vi "write_erg.vi"(8 "error in (no error)":errorcluster, 9 "byte count":u32, 10 "unsigned byte array":u8[](array[numeric]), 11 "VISA resource name":refnum<visa-resource-name>) -> (0 "error out":errorcluster, 1 "Errors":bool, 2 "unsigned byte array 2":u8[](array[numeric]), 3 "VISA resource name out":refnum<visa-resource-name>)   [LabVIEW 2018]
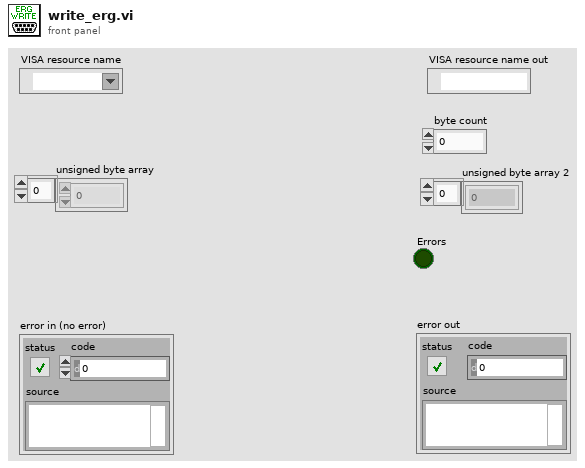
[diagram p1: front panel]
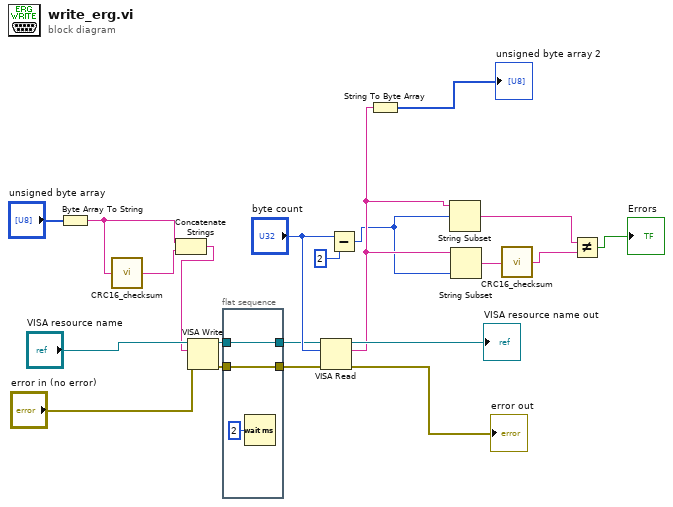
[diagram p0: block diagram]
diagram:
  n1 = Byte Array To String(unsigned byte array="unsigned byte array") -> (string=w17:string)
  n2 = call "CRC16_checksum.vi"("message"=w17) -> ("CRC16"=w16:string)
  n3 = Concatenate Strings(w17, w16) -> (w15:string)
  n4 = VISA Write(VISA resource name="VISA resource name", write buffer=w15, error in (no error)="error in (no error)") -> (VISA resource name out=w4:refnum<visa-resource-name>, error out=w1:errorcluster)  [unwired: 1 out]
  n5 = flat-sequence {
    tunnel: w4 -> [w24]
    tunnel: [w24] -> w3
    tunnel: [w23] -> w2
    tunnel: w1 -> [w23]
    frame #0 {
      n6 = Wait (ms)(milliseconds to wait=u32 2) -> ()  [unwired: 1 out]
    }
  }
  n7 = VISA Read(VISA resource name=w3, byte count="byte count", error in (no error)=w2) -> (VISA resource name out=→"VISA resource name out":refnum<visa-resource-name>, read buffer=w8:string, error out=→"error out":errorcluster)  [unwired: 1 out]
  n8 = Subtract(x="byte count", y=u32 2) -> (x-y=w5:u32)
  n9 = String To Byte Array(string=w8) -> (unsigned byte array=→"unsigned byte array 2":u8[])
  n10 = String Subset(string=w8, offset (0)=w5) -> (substring=w10:string)  [unwired: 1 in]
  n11 = String Subset(string=w8, length (rest)=w5) -> (substring=w12:string)  [unwired: 1 in]
  n12 = call "CRC16_checksum.vi"("message"=w12) -> ("CRC16"=w11:string)
  n13 = Not Equal?(x=w10, y=w11) -> (x != y?=→"Errors":bool)
